vi "Select Instrument.vi"(8 "error in (no error)":errorcluster, 10 "Selected":i32, 11 "Configuration UI in":refnum<class "Configuration UI.lvclass">) -> (0 "error out":errorcluster, 3 "Configuration UI out":refnum<class "Configuration UI.lvclass">)   [LabVIEW 2023, in "Configuration UI.lvlib" / "Configuration UI.lvclass"]
doc: "Using the <b>selected</b> index \n1. Access the configuration keys for the specific device \n2. Write the Key Names and Key Values to the Keys Multicolumn Listbox \n3. Access the signal defintions for the specific device\n4. Write the Signal Headers and Values to the multicolumn listbox"
uses:
  Project/Configuration UI.lvclass
  Project/Configuration UI.lvclass/Configuration UI.ctl
  builds/Tools/Config.lvlibp/Accessors/Write Device.vi
  builds/Tools/Config.lvlibp/Accessors/Read Device Keys.vi
  builds/Tools/Config.lvlibp/Accessors/Read Device Key Values.vi
  builds/Tools/Config.lvlibp/Accessors/Read Device Signals.vi
  builds/Tools/Config.lvlibp/Config.lvclass
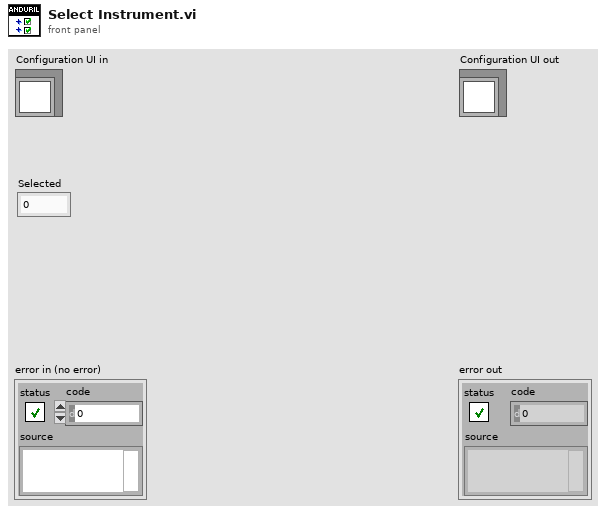
[diagram p1: front panel]
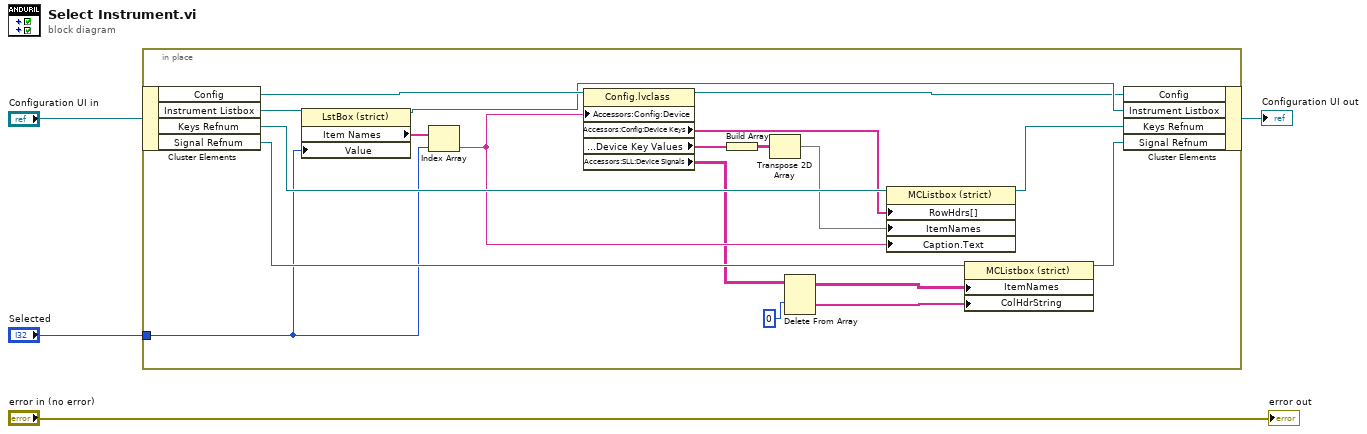
[diagram p0: block diagram]
diagram:
  n1 = in-place {
    in-place-border: "Selected" -> [w6]
    n2 = in-place-cluster #1("Configuration UI in") -> ("Config"=w23:refnum<class "Config.lvclass">, "Instrument Listbox"=w22:refnum<vi>, "Keys Refnum"=w18:refnum<vi>, "Signal Refnum"=w17:refnum<vi>)
    n3 = property class="LstBox (strict)"(reference=w22, "Value"=w6) -> (reference out=w20:refnum<vi>, "Item Names"=w21:string[])  [unwired: 1 in, 1 out]
    n4 = Index Array(array=w21, index=w6) -> (element=w11:string)
    n5 = property class="Config.lvclass"(reference=w23, "Accessors:Config:Device"=w11) -> (reference out=w19:refnum<class "Config.lvclass">, "Accessors:Config:Device Keys"=w5:string[], "Accessors:Config:Device Key Values"=w14:string[], "Accessors:SLL:Device Signals"=w10:string[][])  [unwired: 1 in, 1 out]
    n6 = Build Array(w14) -> (w13:string[][])
    n7 = Transpose 2D Array(2D array=w13) -> (transposed array=w12:string[][])
    n8 = Delete From Array(array=w10, index (row)=0) -> (deleted portion=w7:string[], array with subset deleted=w9:string[][])  [unwired: 2 in]
    n9 = property class="MCListbox (strict)"(reference=w18, "RowHdrs[]"=w5, "ItemNames"=w12, "Caption.Text"=w11) -> (reference out=w16:refnum<vi>)  [unwired: 1 in, 1 out]
    n10 = property class="MCListbox (strict)"(reference=w17, "ItemNames"=w9, "ColHdrString"=w7) -> (reference out=w15:refnum<vi>)  [unwired: 1 in, 1 out]
    n11 = in-place-cluster #1("Config"=w19, "Instrument Listbox"=w20, "Keys Refnum"=w16, "Signal Refnum"=w15) -> (→"Configuration UI out":refnum<class "Configuration UI.lvclass">)
  }
  "error out" <- "error in (no error)"
